vi "Untitled 2.vi"() -> ()   [LabVIEW 2019]
panel:
  out "red":bool
  out "yellow":bool
  out "green":bool
  in  "stop":bool
  out "Numeric":dbl
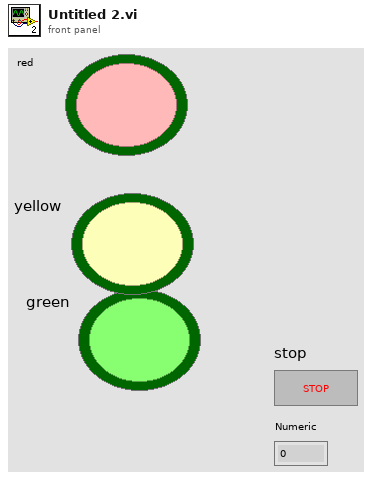
[diagram p1: front panel]
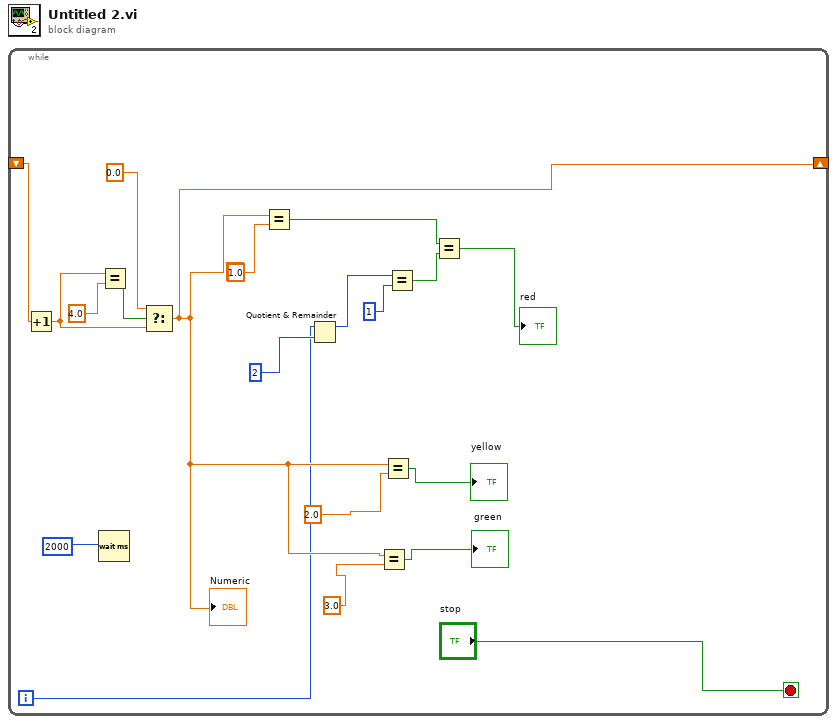
[diagram p0: block diagram]
diagram:
  n1 = while {
    shift-right: [w11] -> _
    shift-left: _ -> [w16]
    i -> [w1]
    stop <- "stop" stop-if-true
    (unwired) 1.0
    n2 = Increment(x=w16) -> (x+1=w6:dbl)
    n3 = Wait (ms)(milliseconds to wait=2000) -> ()  [unwired: 1 out]
    n4 = Equal?(x=w6, y=4.0 ("x")) -> (x = y?=w15:bool)
    n5 = Select(t=0.0, s=w15, f=w6) -> (s? t:f=w11:dbl)
    "Numeric" <- w11
    n6 = Equal?(x=w11, y=1.0) -> (x = y?=w3:bool)
    n7 = Quotient & Remainder(x=w1, y=2) -> (x-y*floor(x/y)=w5:i32)  [unwired: 1 out]
    n8 = Equal?(x=w11, y=3.0) -> (x = y?=→"green":bool)
    n9 = Equal?(x=w11, y=2.0) -> (x = y?=→"yellow":bool)
    n10 = Equal?(x=w5, y=1) -> (x = y?=w4:bool)
    n11 = Equal?(x=w3, y=w4) -> (x = y?=→"red":bool)
  }
